vi "Delay_ms.vi"(8 "error in (no error)":errorcluster caption="에러 입력(에러 없음)", 11 "대기 시간(ms)":u32=2000) -> (0 "error out":errorcluster caption="에러 출력")   [LabVIEW 2015]
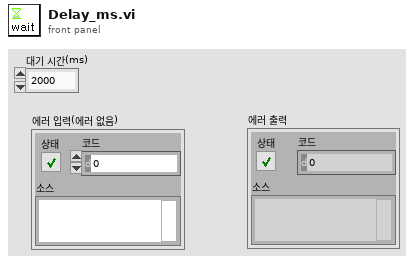
[diagram p1: front panel]
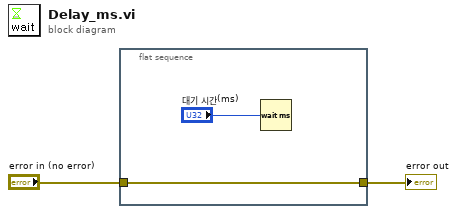
[diagram p0: block diagram]
diagram:
  n1 = flat-sequence {
    tunnel: [w3] -> w2
    tunnel: "error in (no error)" -> [w3]
    frame #0 {
      n2 = Wait (ms)(milliseconds to wait="대기 시간(ms)") -> ()  [unwired: 1 out]
    }
  }
  "error out" <- w2
